vi "CropAndCombineTIFFs.vi"(0 "file path":path) -> ()   [LabVIEW 2011]
uses:
  tiff/TiffModules/AddTiffPage_U16_text_res.vi
panel:
  in  "Save file type":u16(ring)=257 items=["Big-Endian"=0, "Native"=1, "Little-Endian"=2, "BigTiff-Big-Endian"=256, "Bigtiff,Native"=257, "Biftiff,Littleendian"=258]
  in  "Stop at offset:":u64=2147000000
  out "Input-File":i32
  out "AfterDIRoffset":u64 format="%09d"
  out "Files":path[](array[path])
  in  "y-length":i32=1040
  in  "y-start":i32
  in  "x-length":i32=2286
  in  "x-start":i32
  out "Input-page":i32
  out "string":string
  out "xy-resolution":cluster{"x":dbl, "y":dbl}
  out "Out":u16[][](graph)
  out "In":u16[][](graph)
  # "select a tiff file, (all files with @#### will also be used)\nenter crop data run new name with _cropcombine.tif\nstops at last image or tiff-offset 2^31 (or as specified)\nNow works als with bigtif"
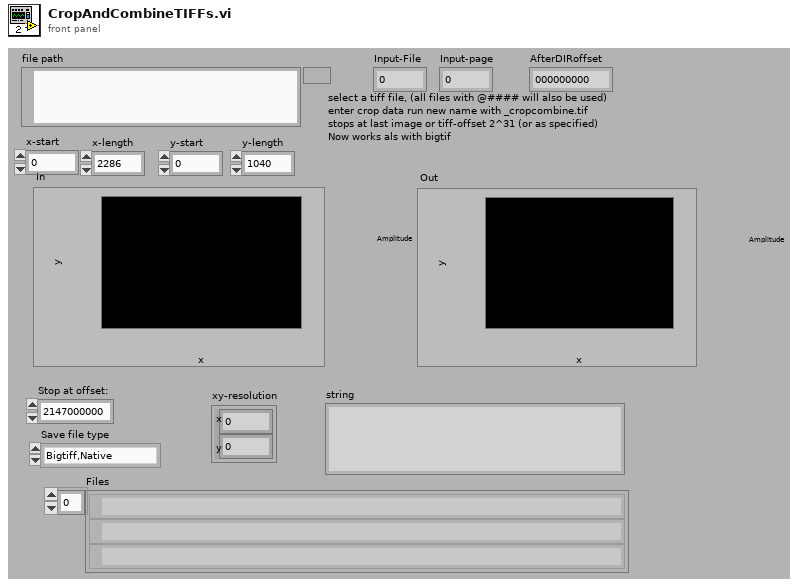
[diagram p1: front panel]
types:
  T1 = cluster{"Tiff refnum":refnum<file>, "BigTiff,Endian":u16}
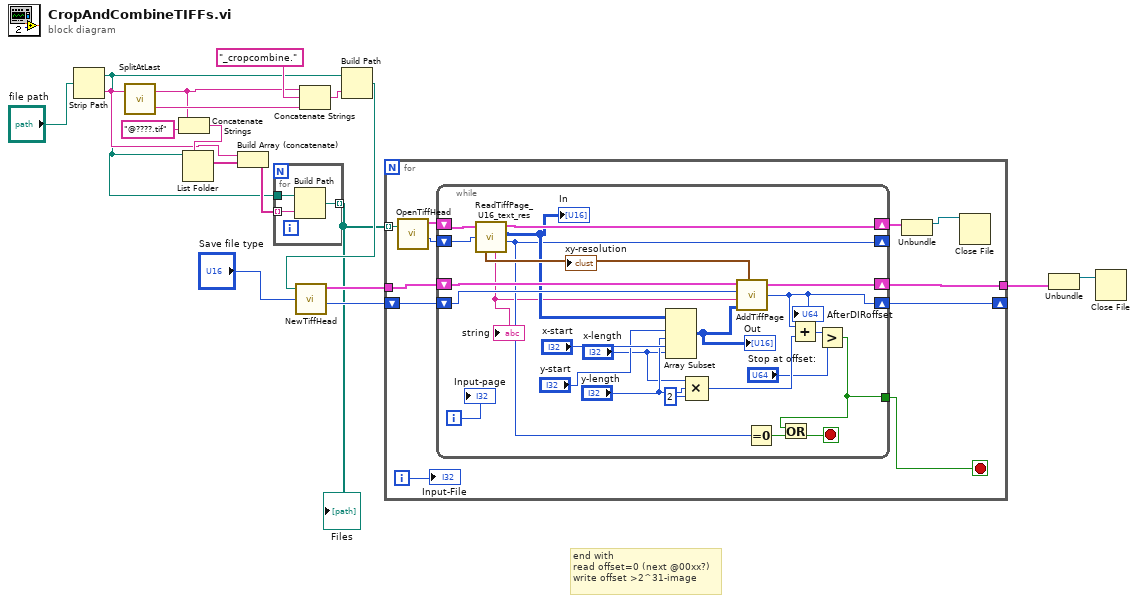
[diagram p0: block diagram]
diagram:
  # "end with \nread offset=0 (next @00xx?)\nwrite offset >2^31-image"
  n1 = Strip Path(path="file path") -> (stripped path=w3:path, name=w5:string)
  n2 = call "SplitAtLast.vi"("In-String"=w5) -> ("end"=w17:string, "Front (default)"=w9:string)  [unwired: 1 in]
  n3 = Concatenate Strings(w9, "@????.tif" ("string")) -> (w7:string)
  n4 = List Folder(path=w3, pattern=w7) -> (filenames=w6:string[])  [unwired: 2 in, 3 out]
  n5 = Build Array (concatenate)(w5, w6) -> (w4:string[])
  n6 = for {
    tunnel: w4 -> [w21] mode=indexing
    tunnel: w3 -> [w20]
    tunnel: [w19] -> w2 mode=indexing
    n7 = Build Path(base path=w20, name or relative path=w21) -> (appended path=w19:path)
  }
  "Files" <- w2
  n8 = Concatenate Strings(w9, "_cropcombine." ("String"), w17) -> (w16:string)
  n9 = Build Path(base path=w3, name or relative path=w16) -> (appended path=w15:path)
  n10 = call "NewTiffHead.vi"("file path"=w15, "BigTiff,Endian"="Save file type") -> ("TIFF file"=w13:T1, "Place for first IFD (8,eof-position)"=w12:u64)  [unwired: 2 in, 1 out]
  n11 = for {
    tunnel: w13 -> [w31]
    tunnel: [w27] -> w11
    tunnel: w2 -> [w25] mode=indexing
    shift-right: [w22] -> _
    shift-left: w12 -> [w29]
    i -> [w23]
    stop <- w24 stop-if-true
    n12 = call "OpenTiffHead.vi"("file path"=w25) -> ("TIFF file"=w32:T1, "first Diroffset"=w30:u64)  [unwired: 2 in, 1 out]
    n13 = while {
      shift-right: [w47] -> w28
      shift-left: w32 -> [w50]
      shift-right: [w55] -> w27
      shift-left: w31 -> [w56]
      shift-right: [w45] -> _
      shift-left: w30 -> [w49]
      shift-right: [w38] -> w22
      shift-left: w29 -> [w54]
      tunnel: [w33] -> w24
      i -> [w52]
      stop <- w34 stop-if-true
      n14 = call "ReadTiffPage_U16_text_res.vi"("TIFF file"=w50, "IFDoffset"=w49) -> ("Pixelsize [µm]"=w48:cluster{"x":dbl, "y":dbl}, "TIFF file out"=w47:T1, "16-bit pixmap"=w46:u16[][], "string"=w44:string, "Next offset"=w45:i64)  [unwired: 3 in, 1 out]
      "In" <- w46
      "xy-resolution" <- w48
      "string" <- w44
      n15 = Array Subset(array=w46, index (row)="y-start", length (row)="y-length", index (col)="x-start", length (col)="x-length") -> (w51:u16[][])
      "Out" <- w51
      n16 = Compound Arithmetic op=MULTIPLY("x-length", "y-length", 2 ("value")) -> (w37:i32)
      n17 = call-poly "AddTiffPage.vi"("TIFF file"=w56, "After last DIROffset"=w54, "Text"=w44, "16-bit pixmap x, y"=w51, "Pixelsize [µm]"=w48) -> ("TIFF file"=w55:T1, "AfterDIRoffset"=w38:u64)  [unwired: 1 out]
      "AfterDIRoffset" <- w38
      n18 = Equal To 0?(x=w45) -> (x = 0?=w53:bool)
      n19 = Add(x=w38, y=w37) -> (x+y=w36:u64)
      n20 = Greater?(x=w36, y="Stop at offset:") -> (0:w33:bool)
      n21 = Or(x=w33, y=w53) -> (x .or. y?=w34:bool)
      "Input-page" <- w52
    }
    n22 = Unbundle(w28) -> ("Tiff refnum"=w26:refnum<file>)  [unwired: 1 out]
    n23 = Close File(refnum=w26) -> ()  [unwired: 1 in, 2 out]
    "Input-File" <- w23
  }
  n24 = Unbundle(w11) -> ("Tiff refnum"=w10:refnum<file>)  [unwired: 1 out]
  n25 = Close File(refnum=w10) -> ()  [unwired: 1 in, 2 out]
